vi "TestGraphUpdating.vi"() -> ()   [LabVIEW 2017]
uses:
  Parameters/ExposeParameterBindingType.ctl
panel:
  in  "DoLogging":bool
  in  "Update count":dbl
  out "TestGraph":dbl[][](graph)
  in  "TestMatrix":dbl[][](array[numeric])
  in  "MatrixUpdateTime":dbl=100.0 caption="MatrixUpdateTime [ms]"
  in  "MatrixSize":dbl=100.0
  out "Flipper":bool
  out "Log":string
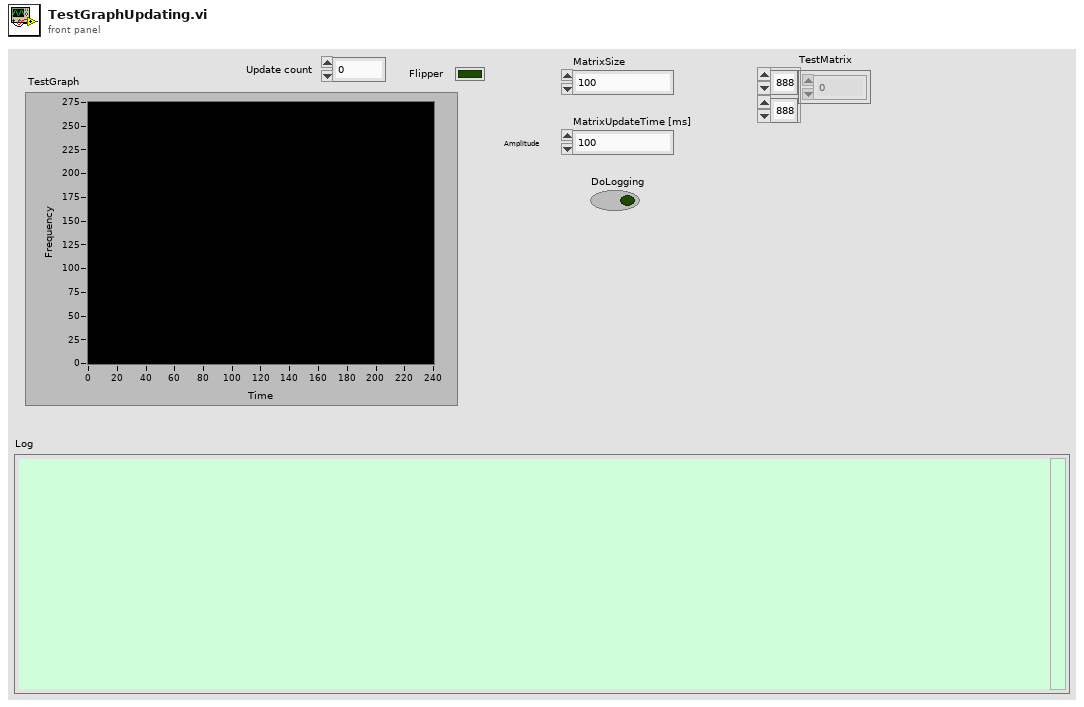
[diagram p1: front panel]
types:
  T1 = typedef "ExposeParameterBindingType.ctl" = enum16{"ToRemote", "FromRemote", "Bidrectional"}
  T2 = typedef "ExposeInfo.ctl" = cluster{"CSCom":refnum<k24>, "URL":string, "Events Category":string, "ID":string}
  T3 = typedef "ExposeEventRegistrationDataType.ctl" = refnum<event-registration>
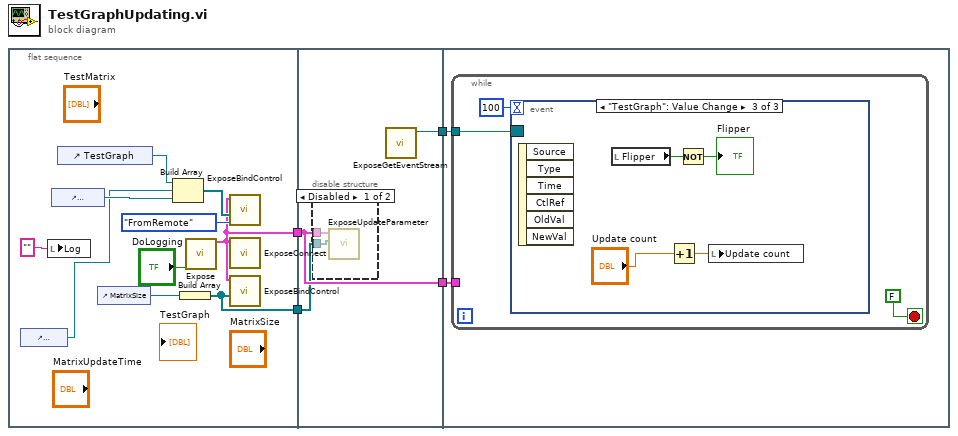
[diagram p0: block diagram]
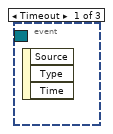
[diagram p3: hidden frame]
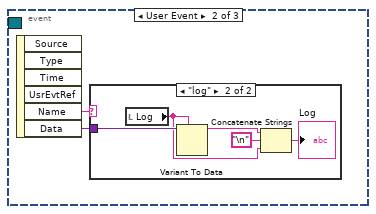
[diagram p4: hidden frame]
diagram:
  n1 = flat-sequence {
    tunnel: [w10] -> w4
    tunnel: [w9] -> w1
    tunnel: w4 -> [w16]
    tunnel: [w16] -> w3
    tunnel: [w17] -> w2
    tunnel: w1 -> [w15]
    tunnel: w3 -> [w21]
    tunnel: w2 -> [w20]
    frame #0 {
      n2 = control-ref of="TestMatrix"() -> (w7:refnum<vi>)
      n3 = local write "Log"("") -> ()
      n4 = control-ref of="MatrixUpdateTime"() -> (w8:refnum<vi>)
      n5 = control-ref of="TestGraph"() -> (w6:refnum<vi>)
      n6 = control-ref of="MatrixSize"() -> (w11:refnum<vi>)
      n7 = Build Array(w6, w7, w8) -> (w12:refnum<vi>[])
      n8 = Build Array(w11) -> (w9:refnum<vi>[])
      n9 = call "Expose.vi"("DoLogging"="DoLogging") -> ("Expose"=w10:T2)  [unwired: 14 in]
      n10 = call "ExposeBindControl.vi"("Binding Type"=ExposeParameterBindingType."FromRemote", "Controls"=w12, "Expose Info"=w10) -> ()  [unwired: 9 in]
      n11 = call "ExposeConnect.vi"("Expose Info"=w10) -> ()  [unwired: 9 in, 2 out]
      n12 = call "ExposeBindControl.vi"("Controls"=w9, "Expose Info"=w10) -> ()  [unwired: 10 in]
    }
    frame #1 {
      n13 = disable-structure shown="Disabled" {
        disable-tunnel: w16 -> [w19 _]
        disable-tunnel: w15 -> [w18 _]
        frame Disabled {
          n14 = call "ExposeUpdateParameter.vi"("Parameter"=w18, "Expose Info"=w19) -> ()  [unwired: 9 in, 1 out]
        }
        frame Enabled {
        }
      }
      n15 = call "ExposeGetEventStream.vi"() -> ("Event Registration Refnum out"=w17:T3)  [unwired: 8 in, 3 out]
    }
    frame #2 {
      n16 = while {
        tunnel: w21 -> [_]
        tunnel: w20 -> [w22]
        stop <- FALSE stop-if-true
        n17 = event shown="[2] \"TestGraph\": Value Change" {
          selector: w22 -> [_ _ _]
          dyn-events: _ -> [_ _ _]
          timeout: 100 -> [_ _ _]
          event Timeout {
            n18 = event-data() -> ()  [unwired: 1 in, 3 out]
          }
          event User Event {
            n19 = event-data() -> ("Name"=w26:string, "Data"=w25:variant)  [unwired: 1 in, 4 out]
            n20 = case shown="\"log\"" w26 {
              tunnel: w25 -> [_ w30]
              frame "False", Default {
              }
              frame "log" {
                n21 = local read "Log"() -> (w29:string)
                n22 = Variant To Data(type=w29, Variant=w30) -> (data=w28:string)  [unwired: 1 in, 1 out]
                n23 = Concatenate Strings(w28, "\n", w29) -> (→"Log":string)
              }
            }
          }
          event "TestGraph": Value Change {
            n24 = event-data() -> ()  [unwired: 1 in, 6 out]
            n25 = local read "Flipper"() -> (w35:bool)
            n26 = Increment(x="Update count") -> (x+1=w32:dbl)
            n27 = Not(x=w35) -> (.not. x?=→"Flipper":bool)
            n28 = local write "Update count"(w32) -> ()
          }
        }
      }
    }
  }
